vi "WiiMote Close.vi"(8 "error in (no error)":errorcluster, 11 "wiimote reference":refnum<k24>) -> (0 "error out":errorcluster)   [LabVIEW 2015]
uses:
  C:/Users/gilled/Downloads/EmbeddedLab_v1.70_Courseware-Kobuki/EmbeddedLab_v1.70_Courseware/Courseware/src/LabVIEW/WiiMote/Dependencies/WiimoteLib.dll
  Dependencies/WiimoteLib.dll
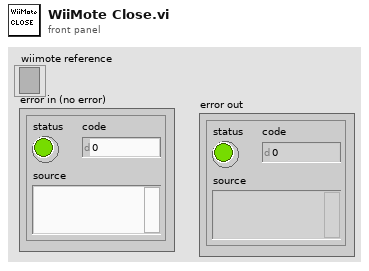
[diagram p1: front panel]
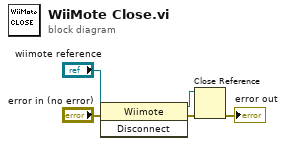
[diagram p0: block diagram]
diagram:
  n1 = invoke class="Wiimote" method="Disconnect"(reference="wiimote reference", error in="error in (no error)") -> (reference out=w5:refnum<k24>, error out=w4:errorcluster)  [unwired: 1 in, 1 out]
  n2 = Close Reference(reference=w5, error in (no error)=w4) -> (error out=→"error out":errorcluster)
